vi "demo1.vi"() -> ()   [LabVIEW 2022 SP3]
panel:
  in  "停止":bool
  out "波形图":dynamicdata(graph)
  in  "噪声频率":dbl(knob) scale=0.0..10.0
  in  "信号频率":dbl(knob) scale=0.0..100.0
  in  "信号幅值":dbl(knob) scale=0.0..10.0
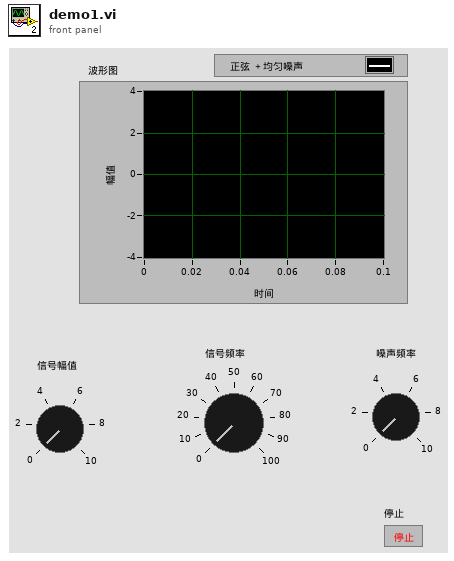
[diagram p1: front panel]
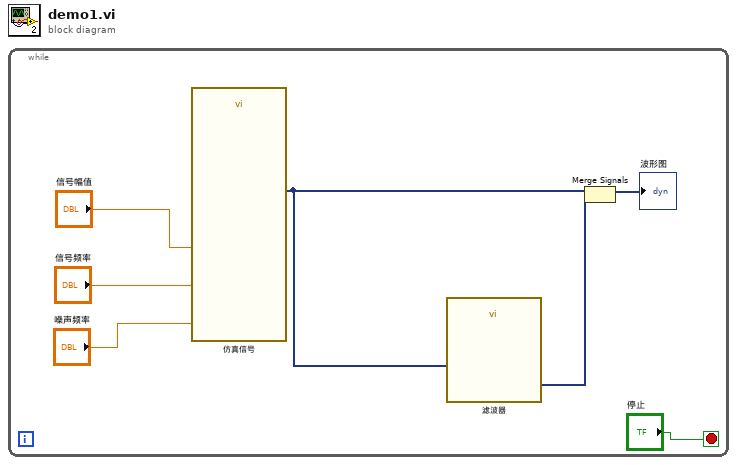
[diagram p0: block diagram]
diagram:
  n1 = while {
    stop <- "停止" stop-if-true
    n2 = call "仿真信号"("Frequency"="信号频率", "Amplitude"="信号幅值", "噪声幅值"="噪声频率") -> ("正弦与均匀噪声"=w4:dynamicdata)  [unwired: 11 in, 1 out]
    n3 = call "滤波器"("Signal"=w4) -> ("Filtered Signal"=w2:dynamicdata)  [unwired: 9 in, 1 out]
    n4 = Merge Signals(w4, w2) -> (→"波形图":dynamicdata)
  }
